vi "fgv_Gslam_edge.vi"(7 "cmd":T4, 11 "edge":T1={"e"=[[2.580150395955859], [1.5130174898420874], [0.0]], "omega"=[[49.99999999999999, 5.513470628566557e-16, 0.0], [2.694565958079997e-16, 49.99999999999999, 0.0], [-0.0, -0.0, 1641.403175005872]], "d1"=8.23607135919321, "d2"=8.243984798861625, "yaw1"=0.0, "yaw2"=0.1963643369696882, "angle1"=-0.44496493256133884, "angle2"=-0.44541413563220067, "id1"=0, "id2"=1}) -> (3 "edge arr":T3(array[cluster]))   [LabVIEW 2019]
uses:
  Ctrl/cmd_ini-add-read.ctl
  <vilib>/Analysis/Matrix/Datatypes/RealMatrix.ctl
  Ctrl/slam_edge.ctl
  <vilib>/Analysis/Matrix/NI_Matrix.lvlib
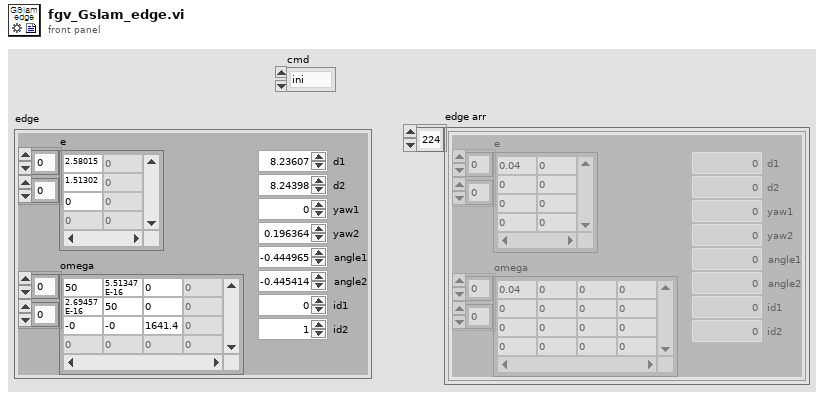
[diagram p1: front panel]
types:
  T1 = typedef "slam_edge.ctl" = cluster{"e":T2, "omega":T2, "d1":dbl, "d2":dbl, "yaw1":dbl, "yaw2":dbl, "angle1":dbl, "angle2":dbl, "id1":i32, "id2":i32}
  T2 = typedef "NI_Matrix.lvlib/RealMatrix.ctl" = dbl[][]
  T3 = cluster{"e":T2, "omega":T2, "d1":dbl, "d2":dbl, "yaw1":dbl, "yaw2":dbl, "angle1":dbl, "angle2":dbl, "id1":i32, "id2":i32}[]
  T4 = typedef "cmd_ini-add-read.ctl" = enum16{"ini", "add", "read"}
  T5 = cluster{"e":T2, "omega":T2, "d1":dbl, "d2":dbl, "yaw1":dbl, "yaw2":dbl, "angle1":dbl, "angle2":dbl, "id1":i32, "id2":i32}
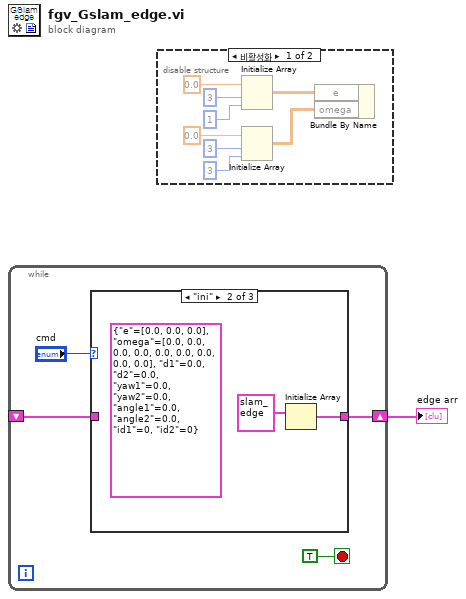
[diagram p0: block diagram]
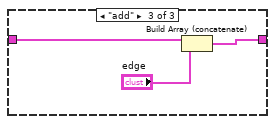
[diagram p4: hidden frame]
diagram:
  n1 = while {
    shift-right: [w4] -> w1
    shift-left: _ -> [w3]
    stop <- TRUE stop-if-true
    n2 = case shown="\"ini\"" "cmd" {
      tunnel: [w6 w8 w10] -> w4
      tunnel: w3 -> [w6 _ w11]
      frame "read", Default {
      }
      frame "ini" {
        (unwired) T5 {"e"=[[0.0], [0.0], [0.0]], "omega"=[[0.0, 0.0, 0.0], [0.0, 0.0, 0.0], [0.0, 0.0, 0.0]], "d1"=0.0, "d2"=0.0, "yaw1"=0.0, "yaw2"=0.0, "angle1"=0.0, "angle2"=0.0, "id1"=0, "id2"=0} ("pf-val")
        n3 = Initialize Array(T1 {"e"=[[2.580150395955859], [1.5130174898420874], [0.0]], "omega"=[[49.99999999999999, 5.513470628566557e-16, 0.0], [2.694565958079997e-16, 49.99999999999999, 0.0], [-0.0, -0.0, 1641.403175005872]], "d1"=8.23607135919321, "d2"=8.243984798861625, "yaw1"=0.0, "yaw2"=0.1963643369696882, "angle1"=-0.44496493256133884, "angle2"=-0.44541413563220067, "id1"=0, "id2"=1} ("pf-val out")) -> (w8:T1[])  [unwired: 1 in]
      }
      frame "add" {
        n4 = Build Array (concatenate)(w11, "edge") -> (w10:T1[])
      }
    }
  }
  "edge arr" <- w1
  n5 = disable-structure shown="비활성화" {
    frame Disabled {
      n6 = Initialize Array(0.0 ("원소"), 3 ("차원 크기"), 1 ("차원 크기")) -> (w13:dbl[][])
      n7 = Initialize Array(0.0 ("원소"), 3 ("차원 크기"), 3 ("차원 크기")) -> (w12:dbl[][])
      n8 = Bundle By Name("e"=w13, "omega"=w12) -> ()  [unwired: 1 in, 1 out]
    }
    frame Enabled {
    }
  }
